vi "configuration UI.vi"() -> ()   [LabVIEW 2013, in "CVT editor node.lvclass"]
uses:
  CVT editor node.lvclass
  <vilib>/CEF_TreeControl/Node/NodeRef.ctl
  <vilib>/CEF_TreeControl/Node/NISE_CEF_Node.lvclass
  <vilib>/NI/AMC/Message Queue.ctl
  <vilib>/NI/AMC/Message.ctl
  <vilib>/NI/Tools/Keyed Array/KeyedArray.ctl
  <vilib>/CEF_TreeControl/Node/UserEventRef.ctl
  <vilib>/CEF_TreeControl/Controls/EventCluster.ctl
  <vilib>/NI/TBM Modules/CVT Access/module/configuration/CVT configuration.lvclass
  <vilib>/NI/Module Execution Interface/Engine Configuration/engine configuration.lvclass
  <vilib>/NI/Tag Bus Data Framework/Configuration Editor/Classes/Engine Parent/Engine Parent Editor Node.lvclass
  <vilib>/NI/Tag Bus/tag/tag descriptor.lvclass
  <vilib>/NI/Tag Bus/tag/Data Type.ctl
  <vilib>/NI/Tag Bus/tag/tag descriptor.lvclass/tag descriptor.ctl
  <vilib>/NI/Tag Bus Module Framework/root configuration/TBM configuration.lvclass/TBM configuration.ctl
  <vilib>/NI/Tag Bus Module Framework/channel/channel classification.ctl
  <vilib>/NI/Tag Bus/tag/write tag name.vi
  <vilib>/NI/Tag Bus/tag/write data type.vi
  <vilib>/NI/Tag Bus Module Framework/root configuration/Read instance name.vi
  <vilib>/NI/Tag Bus Data Framework/Configuration Editor/Classes/Engine Parent/read engine configuration.vi
  <vilib>/NI/Tag Bus Data Framework/Configuration Editor/Classes/Module editor node/Read Module Configuration.vi
  <vilib>/NI/Tag Bus Module Framework/root configuration/create GUID.vi
  <vilib>/NI/Tag Bus Module Framework/root configuration/TBM configuration.lvclass
  <vilib>/NI/Tag Bus Module Framework/module configuration/TBM module configuration.lvclass
  <vilib>/NI/Tag Bus Data Framework/Configuration Editor/Classes/Module editor node/module editor node.lvclass
  <vilib>/CEF_TreeControl/NISE_CEF_TreeControl.lvlib
  <vilib>/NI/Tag Bus Module Framework/channel/TBM channel.lvclass
  <vilib>/NI/Tools/Keyed Array/Tools_KeyedArray.lvlib
  <vilib>/NI/AMC/AMC.lvlib
panel:
  in  "Tab Control":enum32{"Channel Mapping"}(tab)
  in  "Direction":enum32{"From CVT", "To CVT"}(radio)
  in  "remove to":bool
  in  "add to":bool
  in  "remove from":bool
  in  "add from":bool
  in  "toCVTlist":i32(listbox)
  in  "fromCVTlist":i32(listbox)
  in  "avail tags":i32(listbox)=-1
  in  "user event":T1
  in  "main queue":T2
  in  "node ref":T3
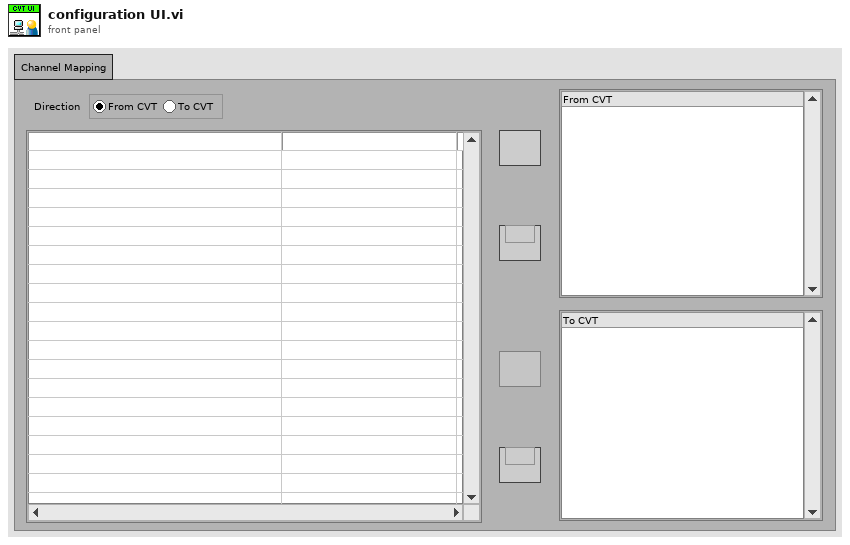
[diagram p1: front panel]
types:
  T1 = typedef "NISE_CEF_Node.lvclass/UserEventRef.ctl" = refnum<user-event>
  T2 = typedef "AMC.lvlib/Message Queue.ctl" = refnum<queue>
  T3 = typedef "NISE_CEF_Node.lvclass/NodeRef.ctl" = refnum<data-value>
  T4 = typedef "tag bus.lvlib/tag descriptor.lvclass/Data Type.ctl" = enum16{"Double", "Single", "I64", "I32", "I16", "I8", "U64", "U32", "U16", "U8", "Boolean", "String", "Array of Double", "Array of Single", "Array of I64", "Array of I32", "Array of I16", "Array of I8", "Array of U64", "Array of U32", "Array of U16", "Array of U8", "Array of Boolean", "Array of String"}
  T5 = typedef "NISE_CEF_TreeControl.lvlib/EventCluster.ctl" = cluster{"command":string, "data":string}
  T6 = typedef "TBM channel.lvclass/channel classification.ctl" = enum16{"input data", "output data", "processing parameter", "processing result"}
  T7 = enum8{"Enabled", "Disabled", "Disabled and Grayed Out"}
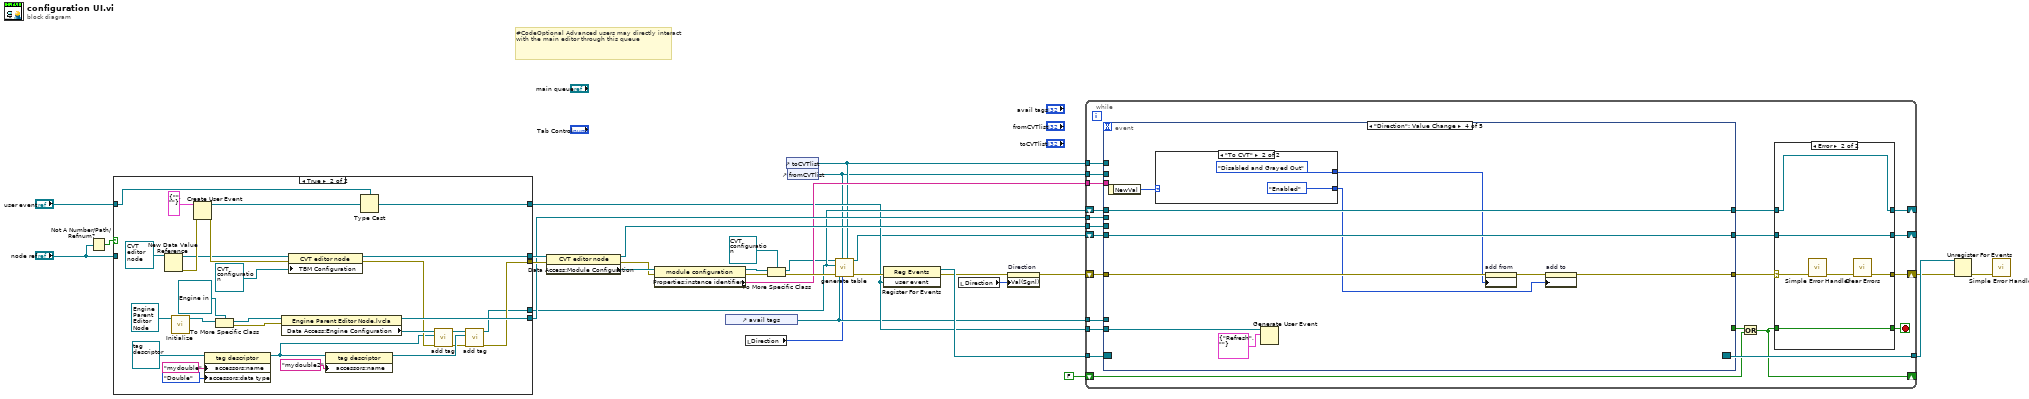
[diagram p0: block diagram]
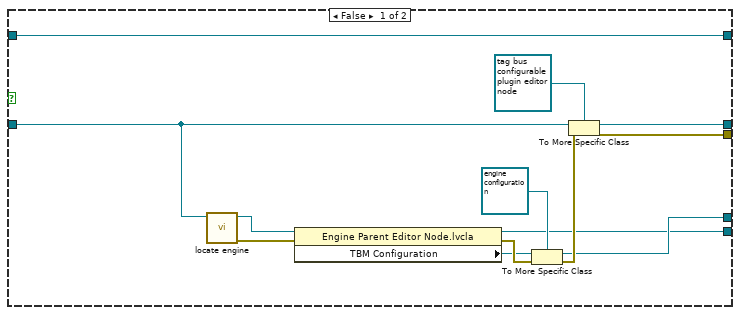
[diagram p2: hidden frame]
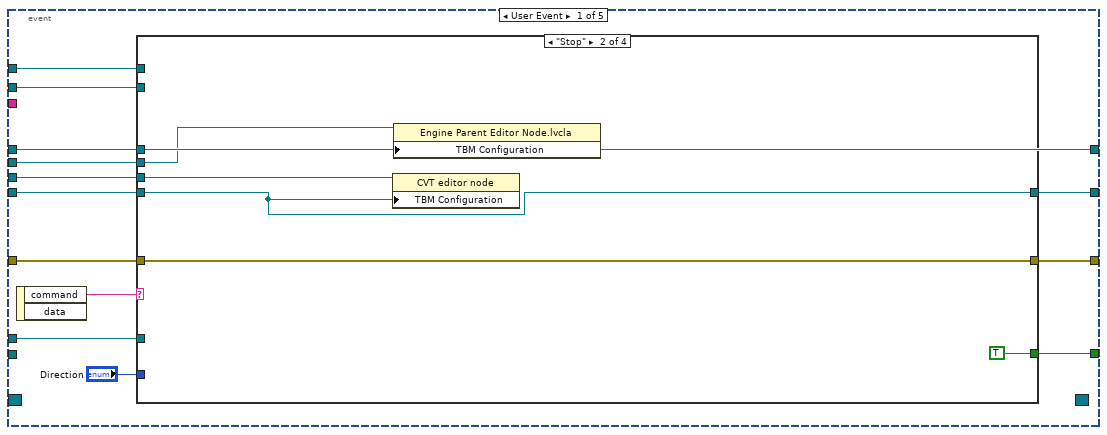
[diagram p4: hidden frame]
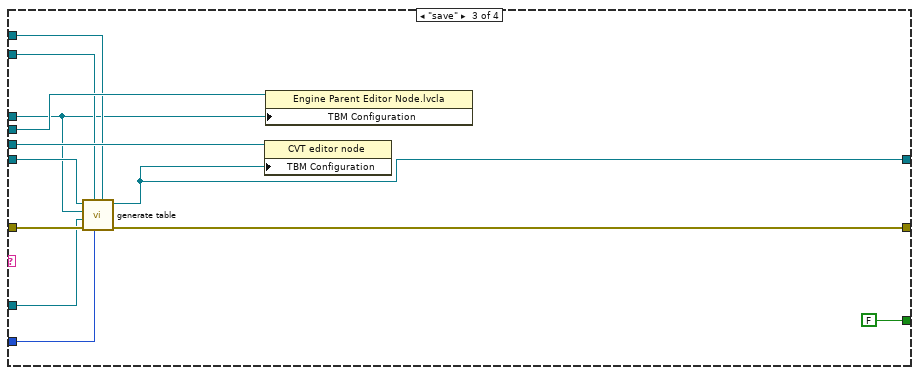
[diagram p6: hidden frame]
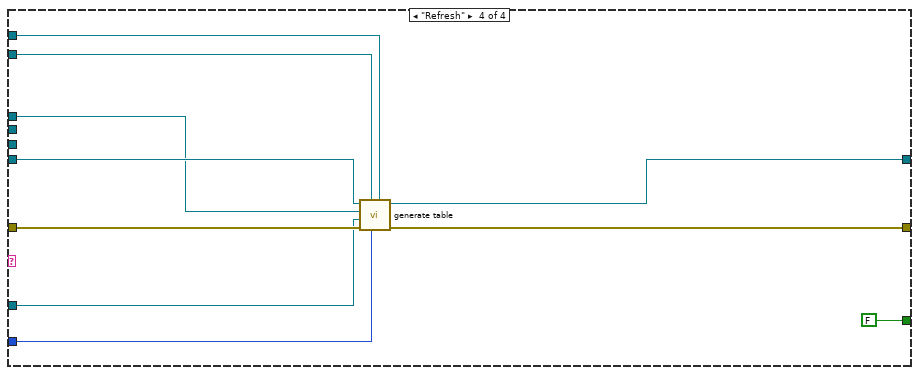
[diagram p7: hidden frame]
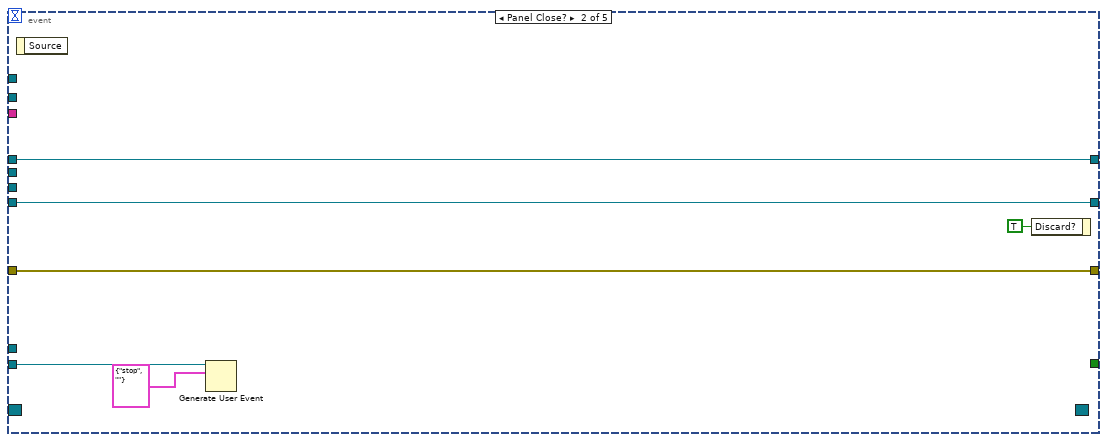
[diagram p8: hidden frame]
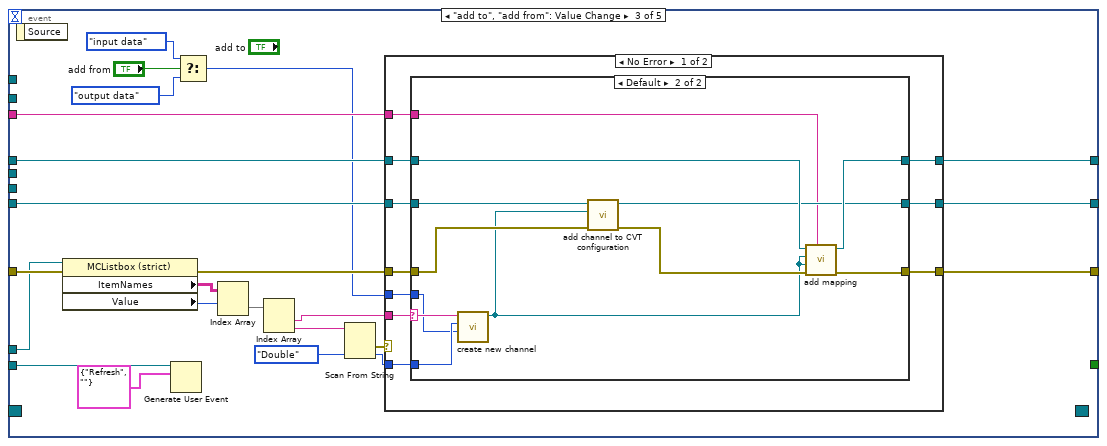
[diagram p9: hidden frame]
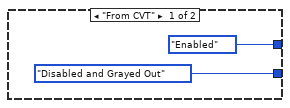
[diagram p12: hidden frame]
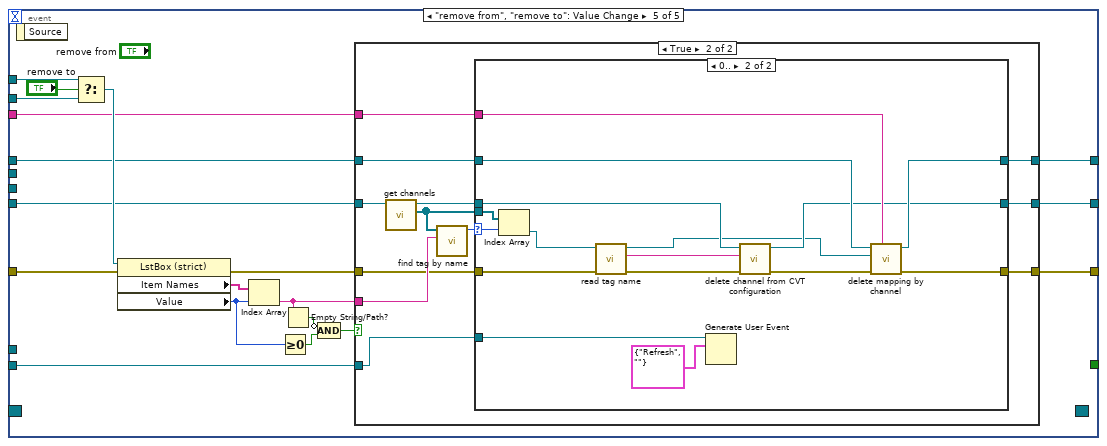
[diagram p13: hidden frame]
diagram:
  # "#CodeOptional Advanced users may directly interact with the main editor through this queue"
  n1 = Not A Number/Path/Refnum?(number/path/refnum="node ref") -> (NaN/Path/Refnum?=w26:bool)
  n2 = case shown="True" w26 {
    tunnel: "user event" -> [w44 w47]
    tunnel: [w44 w48] -> w9
    tunnel: "node ref" -> [w42 _]
    tunnel: [w41 w68] -> w21
    tunnel: [w40 w58] -> w20
    tunnel: [w33 w57] -> w12
    tunnel: [w32 w65] -> w13
    frame False {
      n3 = call <vilib>:"locate engine.vi"("component"=w42) -> ("error out"=w37:errorcluster, "engine"=w39:refnum<data-value>)  [unwired: 9 in]
      n4 = property class="Engine Parent Editor Node.lvcla"(reference=w39, error in=w37) -> (reference out=w32:refnum<data-value>, error out=w36:errorcluster, "TBM Configuration"=w35:refnum<class "TBM configuration.lvclass">)
      n5 = To More Specific Class(target class=refnum<class "engine configuration.lvclass"> refnum ("engine configuration.lvclass"), reference=w35, error in=w36) -> (specific class reference=w33:refnum<class "engine configuration.lvclass">, error out=w34:errorcluster)
      n6 = To More Specific Class(target class=refnum<data-value> refnum ("data value reference"), reference=w42, error in=w34) -> (specific class reference=w41:refnum<data-value>, error out=w40:errorcluster)
    }
    frame True {
      n7 = New Data Value Reference(data value=refnum<class "CVT editor node.lvclass"> refnum ("tag bus configurable plugin editor node")) -> (data value reference=w67:refnum<data-value>, error out=w70:errorcluster)  [unwired: 1 in]
      n8 = call-dynamic "Initialize.vi"("Engine in"=refnum<class "Engine Parent Editor Node.lvclass"> refnum) -> ("data value reference"=w52:T3)  [unwired: 8 in, 2 out]
      n9 = Create User Event(user event datatype=T5 {"command"="", "data"=""} ("event data"), error in=w70) -> (user event=w71:refnum<user-event>, error out=w69:errorcluster)
      n10 = property class="tag descriptor"(reference=refnum<class "tag descriptor.lvclass"> refnum ("tag descriptor"), "accessors:name"="mydouble" ("name"), "accessors:data type"=Data_Type."Double" ("data type")) -> (reference out=w55:refnum<class "tag descriptor.lvclass">)  [unwired: 1 in, 1 out]
      n11 = To More Specific Class(target class=refnum<data-value> refnum ("data value reference"), reference=w52) -> (specific class reference=w51:refnum<data-value>, error out=w49:errorcluster)  [unwired: 1 in]
      n12 = property class="Engine Parent Editor Node.lvcla"(reference=w51, error in=w49) -> (reference out=w65:refnum<data-value>, "Data Access:Engine Configuration"=w64:refnum<class "engine configuration.lvclass">)  [unwired: 1 out]
      n13 = property class="CVT editor node"(reference=w67, error in=w69, "TBM Configuration"=refnum<class "CVT configuration.lvclass"> refnum ("CVT configuration")) -> (reference out=w68:refnum<data-value>, error out=w60:errorcluster)
      n14 = property class="tag descriptor"(reference=w55, "accessors:name"="mydouble2" ("name")) -> (reference out=w56:refnum<class "tag descriptor.lvclass">)  [unwired: 1 in, 1 out]
      n15 = Type Cast(type=w47, x=w71) -> (*(type *) &x=w48:T1)
      n16 = call <vilib>:"add tag.vi"("error in"=w60, "tag descriptor"=w55, "engine configuration in"=w64) -> ("error out"=w46:errorcluster, "engine configuration out"=w45:refnum<class "engine configuration.lvclass">)  [unwired: 7 in]
      n17 = call <vilib>:"add tag.vi"("error in"=w46, "tag descriptor"=w56, "engine configuration in"=w45) -> ("error out"=w58:errorcluster, "engine configuration out"=w57:refnum<class "engine configuration.lvclass">)  [unwired: 7 in]
    }
  }
  n18 = property class="CVT editor node"(reference=w21, error in=w20) -> (reference out=w14:refnum<data-value>, error out=w22:errorcluster, "Data Access:Module Configuration"=w23:refnum<class "TBM module configuration.lvclass">)
  n19 = property class="module configuration"(reference=w23, error in=w22) -> (reference out=w18:refnum<class "TBM module configuration.lvclass">, error out=w19:errorcluster, "Properties:instance identifier"=w11:string)
  n20 = control-ref of="avail tags"() -> (w8:refnum<vi>)
  n21 = local read "Direction"() -> (w1:enum32{"From CVT", "To CVT"})
  n22 = To More Specific Class(target class=refnum<class "CVT configuration.lvclass"> refnum ("CVT configuration"), reference=w18, error in=w19) -> (specific class reference=w10:refnum<class "CVT configuration.lvclass">, error out=w16:errorcluster)
  n23 = control-ref of="toCVTlist"() -> (w7:refnum<vi>)
  n24 = control-ref of="fromCVTlist"() -> (w6:refnum<vi>)
  n25 = call "generate table.vi"("to cvt"=w7, "Direction"=w1, "from cvt"=w6, "error in"=w16, "avail tags"=w8, "engine configuration in"=w12, "cvt in"=w10) -> ("error out"=w27:errorcluster, "cvt out"=w5:refnum<class "CVT configuration.lvclass">)  [unwired: 3 in]
  n26 = register-events(error in=w27, w9) -> (reference out=w31:refnum<event-registration>, error out=w4:errorcluster)  [unwired: 1 in]
  n27 = local read "Direction"() -> (w2:enum32{"From CVT", "To CVT"})
  n28 = property on="Direction" class="RadioBtnsControl (strict)"(error in=w4, "Val(Sgnl)"=w2) -> (error out=w3:errorcluster)  [unwired: 1 in, 1 out]
  n29 = while {
    tunnel: w31 -> [w94]
    tunnel: [w93] -> w30
    shift-right: [w86] -> w29
    shift-left: w3 -> [w92]
    shift-right: [w88] -> _
    shift-left: FALSE -> [w87]
    shift-right: [w83] -> _
    shift-left: w5 -> [w85]
    tunnel: w11 -> [w82]
    shift-right: [w79] -> _
    shift-left: w12 -> [w81]
    tunnel: w14 -> [w78]
    tunnel: w13 -> [w77]
    tunnel: w9 -> [w76]
    tunnel: w8 -> [w75]
    tunnel: w7 -> [w74]
    tunnel: w6 -> [w73]
    stop <- w90 stop-if-true
    n30 = event shown="[3] \"Direction\": Value Change" {
      selector: w94 -> [_ _ _ _ _]
      dyn-events: [_ _ _ _ _] -> w93
      timeout: _ -> [_ _ _ _ _]
      tunnel: [w117 _ _ _ _] -> w89
      tunnel: [w114 w153 w175 w208 w226] -> w91
      tunnel: w92 -> [w115 w153 w176 w210 w234]
      tunnel: w85 -> [w113 w152 w169 w214 w225]
      tunnel: [w109 w152 w170 w214 w224] -> w84
      tunnel: w82 -> [_ _ w174 _ w219]
      tunnel: w81 -> [w111 w151 w168 w213 w222]
      tunnel: [w111 w151 w171 w213 w223] -> w80
      tunnel: w78 -> [w112 _ _ _ _]
      tunnel: w77 -> [w110 _ _ _ _]
      tunnel: w76 -> [_ w148 w173 w211 w221]
      tunnel: w75 -> [w108 _ w163 _ _]
      tunnel: w74 -> [w107 _ _ _ w236]
      tunnel: w73 -> [w106 _ _ _ w237]
      event User Event {
        n31 = event-data() -> ("command"=w116:string)  [unwired: 1 in, 1 out]
        n32 = case shown="\"Stop\"" w116 {
          tunnel: [_ TRUE FALSE FALSE] -> w117
          tunnel: w115 -> [w119 w124 w134 w146]
          tunnel: [w119 w124 w133 w145] -> w114
          tunnel: w113 -> [w118 w123 w132 w144]
          tunnel: w112 -> [_ w122 w136 _]
          tunnel: w111 -> [_ w121 w128 w143]
          tunnel: w110 -> [_ w120 w135 _]
          tunnel: [w118 w123 w131 w142] -> w109
          tunnel: w108 -> [_ _ w127 w141]
          tunnel: w107 -> [_ _ w130 w140]
          tunnel: w106 -> [_ _ w129 w139]
          tunnel: "Direction" -> [_ _ w126 w138]
          frame Default {
          }
          frame "Stop" {
            n33 = property class="CVT editor node"(reference=w122, "TBM Configuration"=w123) -> ()  [unwired: 1 in, 2 out]
            n34 = property class="Engine Parent Editor Node.lvcla"(reference=w120, "TBM Configuration"=w121) -> ()  [unwired: 1 in, 2 out]
          }
          frame "save" {
            n35 = call "generate table.vi"("to cvt"=w130, "Direction"=w126, "from cvt"=w129, "error in"=w134, "avail tags"=w127, "engine configuration in"=w128, "cvt in"=w132) -> ("error out"=w133:errorcluster, "cvt out"=w131:refnum<class "CVT configuration.lvclass">)  [unwired: 3 in]
            n36 = property class="CVT editor node"(reference=w136, "TBM Configuration"=w131) -> ()  [unwired: 1 in, 2 out]
            n37 = property class="Engine Parent Editor Node.lvcla"(reference=w135, "TBM Configuration"=w128) -> ()  [unwired: 1 in, 2 out]
          }
          frame "Refresh" {
            n38 = call "generate table.vi"("to cvt"=w140, "Direction"=w138, "from cvt"=w139, "error in"=w146, "avail tags"=w141, "engine configuration in"=w143, "cvt in"=w144) -> ("error out"=w145:errorcluster, "cvt out"=w142:refnum<class "CVT configuration.lvclass">)  [unwired: 3 in]
          }
        }
      }
      event Panel Close? {
        n39 = event-data() -> ()  [unwired: 1 in, 1 out]
        n40 = Generate User Event(user event=w148, event data cluster=T5 {"command"="stop", "data"=""} ("event data")) -> ()  [unwired: 2 in, 2 out]
        n41 = event-data("Discard?"=TRUE) -> ()  [unwired: 1 in, 1 out]
      }
      event "add to", "add from": Value Change {
        n42 = event-data() -> ()  [unwired: 1 in, 1 out]
        n43 = property class="MCListbox (strict)"(reference=w163, error in=w176) -> (error out=w164:errorcluster, "ItemNames"=w162:string[][], "Value"=w161:i32)  [unwired: 1 out]
        n44 = Generate User Event(user event=w173, event data cluster=T5 {"command"="Refresh", "data"=""} ("event data")) -> ()  [unwired: 2 in, 2 out]
        n45 = Select(t=channel_classification."input data" ("channel classification"), s="add from", f=channel_classification."output data" ("channel classification")) -> (s? t:f=w154:T6)
        n46 = Index Array(array=w162, index (row)=w161) -> (element=w158:string[])  [unwired: 1 in]
        n47 = Index Array(array=w158) -> (element #1=w157:string, element #2=w160:string)  [unwired: 2 in]
        n48 = Scan From String(input string=w160, default 1=Data_Type."Double" ("data type")) -> (error out=w156:errorcluster, output 1=w155:T4)  [unwired: 3 in, 2 out]
        n49 = case shown="No Error" w156 {
          tunnel: [w186 w202] -> w175
          tunnel: w174 -> [w185 _]
          tunnel: [w184 w204] -> w171
          tunnel: [w183 w203] -> w170
          tunnel: w169 -> [w182 w203]
          tunnel: w168 -> [w181 w204]
          tunnel: w164 -> [w180 w202]
          tunnel: w157 -> [w179 _]
          tunnel: w155 -> [w178 _]
          tunnel: w154 -> [w177 _]
          frame No Error {
            n50 = case shown="Default" w179 {
              selector: w179 -> [_ w193]
              tunnel: [w189 w201] -> w186
              tunnel: w180 -> [w189 w196]
              tunnel: w181 -> [w187 w200]
              tunnel: [w188 w197] -> w183
              tunnel: w182 -> [w188 w198]
              tunnel: [w187 w199] -> w184
              tunnel: w185 -> [_ w194]
              tunnel: w178 -> [_ w192]
              tunnel: w177 -> [_ w191]
              frame "" {
              }
              frame Default {
                n51 = call <vilib>:"create new channel.vi"("channel classification"=w191, "data type"=w192, "channel name"=w193) -> ("channel"=w190:refnum<class "TBM channel.lvclass">)  [unwired: 8 in]
                n52 = call <vilib>:"add channel to CVT configuration.vi"("error in"=w196, "channel"=w190, "CVT configuration in"=w198) -> ("error out"=w195:errorcluster, "CVT configuration out"=w197:refnum<class "CVT configuration.lvclass">)  [unwired: 7 in]
                n53 = call <vilib>:"add mapping.vi"("owner ID"=w194, "error in"=w195, "channel"=w190, "tag descriptor"=w190, "engine configuration"=w200) -> ("error out"=w201:errorcluster, "engine configuration out"=w199:refnum<class "engine configuration.lvclass">)  [unwired: 5 in]
              }
            }
          }
          frame Error {
          }
        }
      }
      event "Direction": Value Change {
        n54 = event-data() -> ("NewVal"=w207:enum32{"From CVT", "To CVT"})  [unwired: 1 in]
        n55 = case shown="\"To CVT\"" w207 {
          tunnel: [T7."Enabled" ("Disabled") T7."Disabled and Grayed Out" ("Disabled")] -> w206
          tunnel: [T7."Disabled and Grayed Out" ("Disabled") T7."Enabled" ("Disabled")] -> w205
          frame "From CVT" {
          }
          frame "To CVT" {
          }
        }
        n56 = Generate User Event(user event=w211, event data cluster=T5 {"command"="Refresh", "data"=""} ("event data")) -> ()  [unwired: 2 in, 2 out]
        n57 = property on="add from" class="Bool"(error in=w210, "DisabledEnum"=w206) -> (error out=w209:errorcluster)  [unwired: 1 in, 1 out]
        n58 = property on="add to" class="Bool"(error in=w209, "DisabledEnum"=w205) -> (error out=w208:errorcluster)  [unwired: 1 in, 1 out]
      }
      event "remove from", "remove to": Value Change {
        n59 = event-data() -> ()  [unwired: 1 in, 1 out]
        n60 = Select(t=w236, s="remove to", f=w237) -> (s? t:f=w233:refnum<vi>)
        n61 = property class="LstBox (strict)"(reference=w233, error in=w234) -> (error out=w227:errorcluster, "Item Names"=w232:string[], "Value"=w231:i32)  [unwired: 1 out]
        n62 = Index Array(array=w232, index=w231) -> (element=w220:string)
        n63 = Greater Or Equal To 0?(x=w231) -> (x >= 0?=w229:bool)
        n64 = Empty String/Path?(string/path=w220) -> (empty?=w230:bool)
        n65 = Compound Arithmetic op=AND(invert w230, w229) -> (w228:bool)
        n66 = case shown="True" w228 {
          tunnel: w227 -> [w240 w245]
          tunnel: [w240 w246] -> w226
          tunnel: w225 -> [w239 w251]
          tunnel: [w239 w247] -> w224
          tunnel: [w238 w243] -> w223
          tunnel: w222 -> [w238 w244]
          tunnel: w221 -> [_ w252]
          tunnel: w220 -> [_ w250]
          tunnel: w219 -> [_ w241]
          frame False {
          }
          frame True {
            n67 = call-dynamic "get channels.vi"("CVT configuration in"=w251) -> ("channels"=w242:refnum<class "TBM channel.lvclass">[], "CVT configuration out"=w248:refnum<class "CVT configuration.lvclass">)  [unwired: 9 in]
            n68 = call <vilib>:"find tag by name.vi"("name"=w250, "tags in"=w242) -> ("index"=w249:i32)  [unwired: 9 in]
            n69 = case shown="0.." w249 {
              selector: w249 -> [_ w269]
              tunnel: w252 -> [_ w270]
              tunnel: w248 -> [w255 w267]
              tunnel: [w255 w261] -> w247
              tunnel: [w254 w260] -> w246
              tunnel: w245 -> [w254 w266]
              tunnel: w244 -> [w253 w265]
              tunnel: [w253 w262] -> w243
              tunnel: w242 -> [_ w268]
              tunnel: w241 -> [_ w263]
              frame ..-1 {
              }
              frame 0.. {
                n70 = Index Array(array=w268, index=w269) -> (element=w258:refnum<class "TBM channel.lvclass">)
                n71 = call <vilib>:"read tag name.vi"("error in"=w266, "system tag in"=w258) -> ("error out"=w259:errorcluster, "name"=w256:string, "system tag out"=w257:refnum<class "TBM channel.lvclass">)  [unwired: 7 in]
                n72 = Generate User Event(user event=w270, event data cluster=T5 {"command"="Refresh", "data"=""} ("event data")) -> ()  [unwired: 2 in, 2 out]
                n73 = call <vilib>:"delete channel from CVT configuration.vi"("error in"=w259, "channel to delete"=w256, "CVT configuration in"=w267) -> ("error out"=w264:errorcluster, "CVT configuration out"=w261:refnum<class "CVT configuration.lvclass">)  [unwired: 7 in]
                n74 = call <vilib>:"delete mapping by channel.vi"("owner ID"=w263, "error in"=w264, "channel"=w257, "engine configuration in"=w265) -> ("error out"=w260:errorcluster, "engine configuration out"=w262:refnum<class "engine configuration.lvclass">)  [unwired: 6 in]
              }
            }
          }
        }
      }
    }
    n75 = Or(x=w89, y=w87) -> (x .or. y?=w88:bool)
    n76 = case shown="Error" w91 {
      selector: w91 -> [w97 w103]
      tunnel: [w98 w104] -> w90
      tunnel: w88 -> [w98 w104]
      tunnel: [w97 w101] -> w86
      tunnel: w84 -> [w96 w100]
      tunnel: [w96 w100] -> w83
      tunnel: w80 -> [w95 w99]
      tunnel: [w95 w99] -> w79
      frame No Error {
      }
      frame Error {
        n77 = call <vilib>:"Simple Error Handler.vi"("error in (no error)"=w103) -> ("error out"=w102:errorcluster)  [unwired: 4 in, 4 out]
        n78 = call <vilib>:"Clear Errors.vi"("error in (no error)"=w102) -> ("error out"=w101:errorcluster)  [unwired: 6 in]
      }
    }
  }
  n79 = Unregister For Events(event registration refnum=w30, error in=w29) -> (error out=w15:errorcluster)
  n80 = call <vilib>:"Simple Error Handler.vi"("error in (no error)"=w15) -> ()  [unwired: 4 in, 5 out]
